vi "AlliGator Globals.vi"() -> ()   [LabVIEW 2021, in "AlliGator Globals, Variables & Constants.lvlib"]
doc: "Collects most of AlliGator's global variables (except for some Abort flags and LV2-type global variables)."
uses:
  AlliGator Globals, Variables & Constants.lvlib
panel:
  out "critical bug test":bool
  out "Window Just Opened":bool
  out "About Message":string="Copyright ©2021 National Instruments Corporation. All rights reserved.\nCopyright © 2015-2025 The Regents of University of California\nAuthor: X. Michalet, Department of Chemistry & Biochemistry, UCLA\n\nThis software product was developed using LabVIEW™ and the National Instruments Vision Development and Advanced Analysis Toolkits for LabVIEW. LabVIEW is a trademark of National Instruments and is protected by patents listed at https://www.ni.com/en/about-ni/legal/patents.html\n\nAdditionally, free toolkits distributed by third parties were used in the code development as detailed in the licenses.txt file present in the installation folder.\n\nFunding was provided in part by grants from the US National Institute of Health, US Department of Energy, UC Cancer Research Coordination Committee and the UCLA Jonsson Comprehensive Cancer Center. AlliGator is not endorsed by, or sponsored by any of the above organizations.\n\nThis software is provided without guaranty of any kind, whether expressed or implied. You can redistribute it but not for commercial purpose."
  out "Use IRF-guided Weights":bool
  out "Beta version?":bool
  out "Beta Unlocked?":bool=TRUE
  in  "Alligator Beta Code":string="0.73"
  out "Init (Check Version)":bool
  in  "Alligator version":string="1.02"
  # "1. Make Current Value Default\n2. Save Global VI"
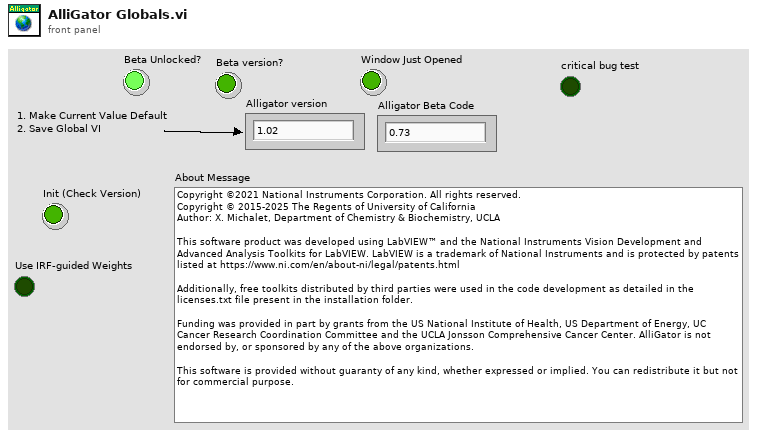
[diagram p1: front panel]
diagram:
